vi "CAN Write.vi"(2 "Error In":errorcluster, 3 "CAN frame":T1 {"payload" format="%x"; "timestamp" format="%<%.7X\n%x>T"; "type" items=["CAN Data"=0, "CAN Remote"=1, "CAN Bus Error"=2, "CAN 2.0 Data"=8, "CAN FD Data"=16, "CAN FD+BRS Data"=24, "J1939 Data"=192, "Delay"=224, "Log Trigger"=225, "Start Trigger"=226]; "identifier" format="%x"}, 4 "Write In":refnum<k21>) -> (0 "Error Out":errorcluster, 1 "Write Out":refnum<k21>)   [LabVIEW 2023]
uses:
  <vilib>/xnet/xnet.llb/XNET Frame CAN.ctl
  <vilib>/xnet/xnet.llb/XNET Frame Type CAN.ctl
  <vilib>/xnet/xnet.llb/XNET Write (Frame CAN).vi
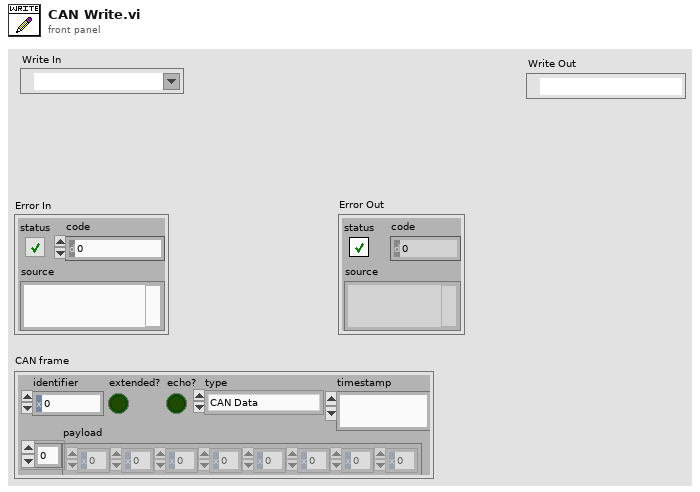
[diagram p1: front panel]
types:
  T1 = typedef "XNET Frame CAN.ctl" = cluster{"timestamp":timestamp, "payload":u8[], "identifier":u32, "type":T2, "extended?":bool, "echo?":bool}
  T2 = typedef "XNET Frame Type CAN.ctl" = u8
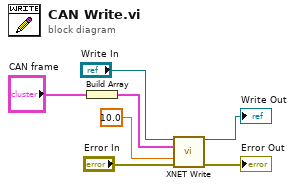
[diagram p0: block diagram]
diagram:
  n1 = Build Array("CAN frame") -> (w6:T1[])
  n2 = call-poly <vilib>:"XNET Write.vi"("session in"="Write In", "data"=w6, "timeout (10)"=10.0, "error in (no error)"="Error In") -> ("session out"=→"Write Out":refnum<k21>, "error out"=→"Error Out":errorcluster)  [unwired: 10 in]
